vi "Clear Gameboard.vi"(8 "error in (no error)":errorcluster, 11 "Buton Refs IN":refnum<vi>[](array[refnum])) -> (0 "error out":errorcluster, 2 "Gameboard":T1)   [LabVIEW 2020]
uses:
  controls/Gameboard Data.ctl
  controls/Player.ctl
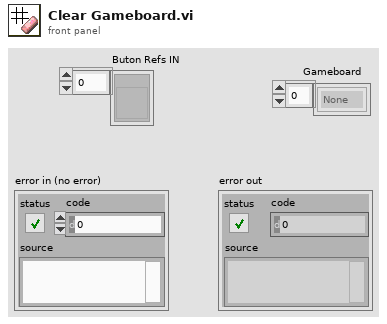
[diagram p1: front panel]
types:
  T1 = typedef "Gameboard Data.ctl" = enum16{"None", "Player 1", "Player 2"}[]
  T2 = typedef "Player.ctl" = enum16{"None", "Player 1", "Player 2"}
  T3 = enum8{"Enabled", "Disabled", "Disabled and Grayed Out"}
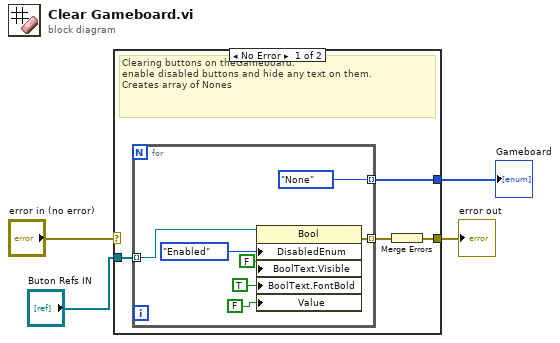
[diagram p0: block diagram]
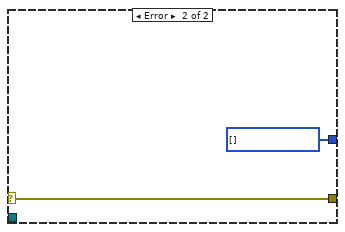
[diagram p2: hidden frame]
diagram:
  n1 = case shown="No Error" "error in (no error)" {
    selector: "error in (no error)" -> [_ w17]
    tunnel: "Buton Refs IN" -> [w8 _]
    tunnel: [w6 w17] -> w2
    tunnel: [w5 w16] -> w1
    frame No Error {
      # "Clearing buttons on theGameboard: \nenable disabled buttons and hide any text on them.\nCreates array of Nones"
      n2 = for {
        tunnel: w8 -> [w15] mode=indexing
        tunnel: [w12] -> w7 mode=indexing
        tunnel: [Player."None" ("Player")] -> w5 mode=indexing
        n3 = property class="Bool"(reference=w15, "DisabledEnum"=T3."Enabled" ("Disabled"), "BoolText.Visible"=FALSE ("Boolean Text.Visible"), "BoolText.FontBold"=TRUE ("Boolean Text.Font:Bold"), "Value"=FALSE) -> (error out=w12:errorcluster)  [unwired: 1 in, 1 out]
      }
      n4 = Merge Errors(w7) -> (w6:errorcluster)
    }
    frame Error {
      w16 = T2[] [] items=["None", "Player 1", "Player 2"]
    }
  }
  "error out" <- w2
  "Gameboard" <- w1
